vi "E Save and close.vi"(0 "Excel._WorkBook":refnum<k7>, 11 "error in (no error)":errorcluster) -> (15 "error out":errorcluster)   [LabVIEW 2009]
doc: "保存表格的改动并关闭表格。"
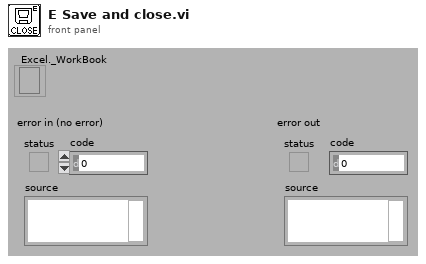
[diagram p1: front panel]
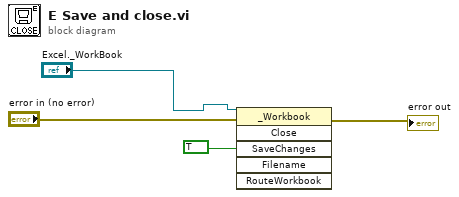
[diagram p0: block diagram]
diagram:
  n1 = invoke class="_Workbook" method="Close"(reference="Excel._WorkBook", error in="error in (no error)", "SaveChanges"=TRUE) -> (error out=→"error out":errorcluster)  [unwired: 3 in, 5 out]
